vi "GUI Main.vi"() -> ()   [LabVIEW 2020]
uses:
  <vilib>/Instr/_visa.llb/VISA Configure Serial Port (Instr).vi
  <vilib>/picture/3D Picture Control/Object/Create Object (name).vi
  <vilib>/picture/3D Picture Control/NI_3D Picture Control.lvlib
panel:
  in  "Resource Name":refnum<visa-resource-name>="COM4"
  in  "Release":bool
  in  "Lock":bool
  in  "Jaw":bool
  in  "Stop":bool
  in  "1":dbl(knob) scale=-30.0..10.0
  in  "2":dbl(knob) scale=-70.0..-15.0
  in  "0":dbl(knob)
  out "Robotic Arm Simulation":refnum<vi>(3d-picture)
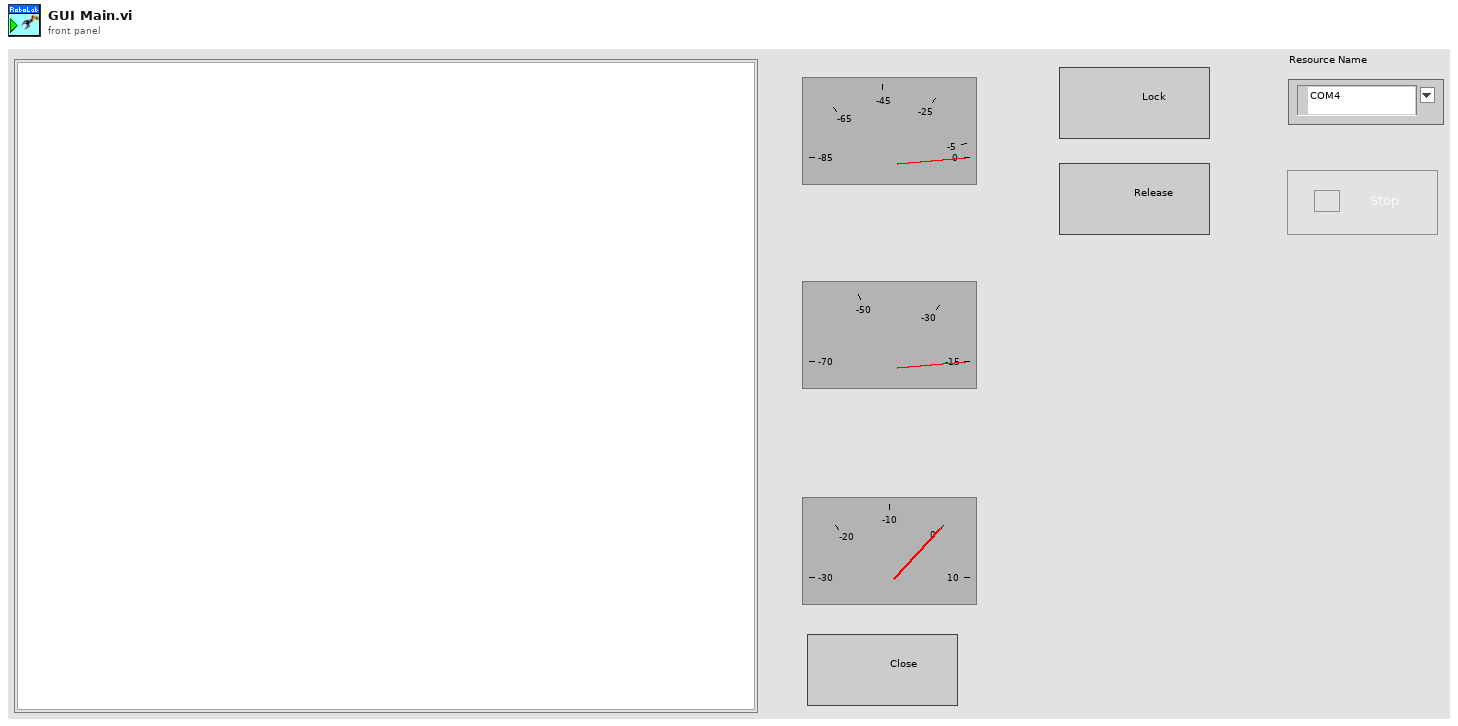
[diagram p1: front panel]
types:
  T1 = cluster{"Red":sgl, "Green":sgl, "Blue":sgl, "Alpha":sgl}
  T2 = cluster{"Name":string, "Parent":string, "Type":enum16{"Joint", "Box", "Cylinder", "Cone", "Sphere", "ASE File", "VRML File", "STL File", "Space"}, "Visible?":bool, "Geometry Definition":dbl[], "Position WRT Parent (X,Y,Z)":dbl[], "Rotation WRT Parent (degrees)":dbl[], "Joint Type":enum16{"Trans_X", "Trans_Y", "Trans_Z", "Rot_X", "Rot_Y", "Rot_Z", "None"}, "Geometry File Path":path, "Indent Level":i32, "Color":u32}[]
  T3 = cluster{"Joint Refnum":refnum<vi>, "Joint Type":enum16{"Trans_X", "Trans_Y", "Trans_Z", "Rot_X", "Rot_Y", "Rot_Z", "None"}, "Position WRT Parent":dbl[], "Rotation WRT Parent":dbl[], "Bar Refnum":refnum<vi>}[]
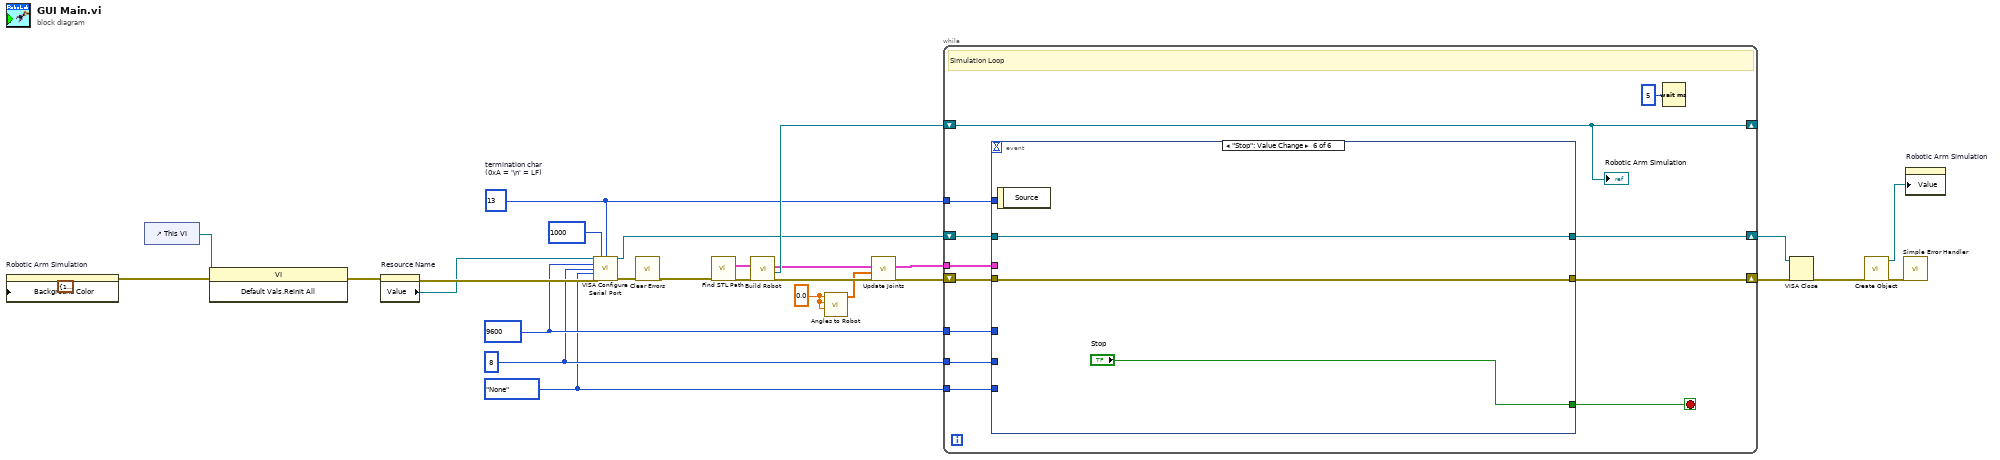
[diagram p0: block diagram]
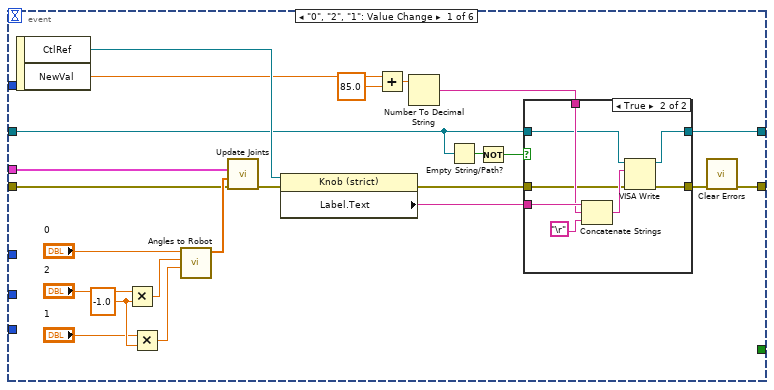
[diagram p2: hidden frame]
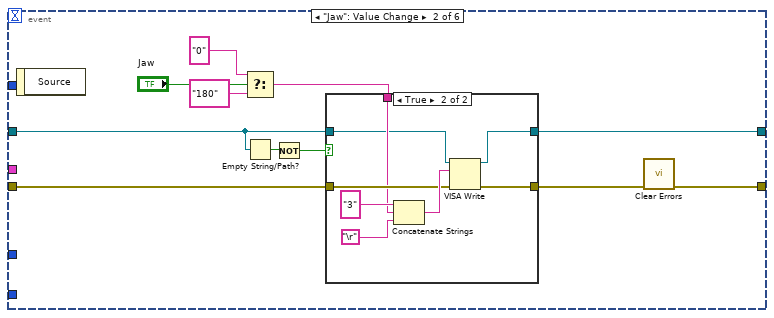
[diagram p4: hidden frame]
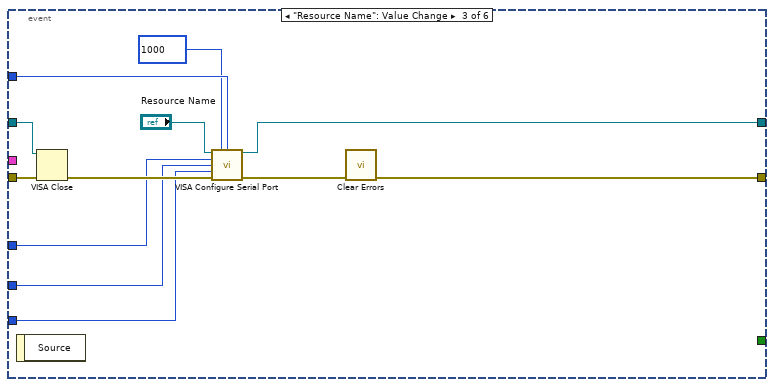
[diagram p6: hidden frame]
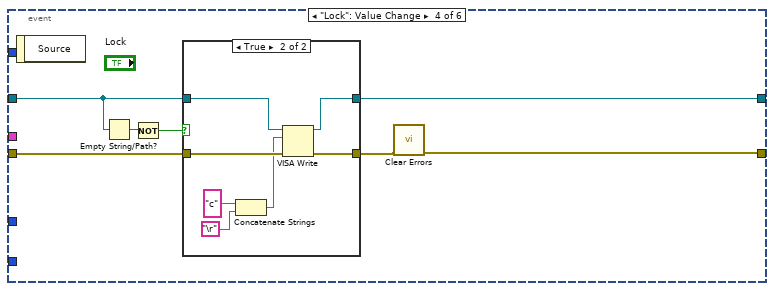
[diagram p7: hidden frame]
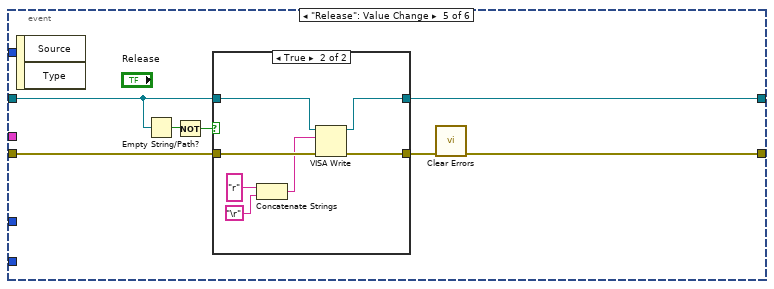
[diagram p9: hidden frame]
diagram:
  w4 = enum16{"None", "Odd", "Even", "Mark", "Space"}."None" ("parity (0:none)")
  w5 = u16 8 ("data bits (8)")
  w6 = u32 9600 ("baud rate (9600)")
  w7 = u8 13  # termination char (0xA = '\n' = LF)
  w18 = 0.0 ("Joint 0")
  n1 = property on="Robotic Arm Simulation" class="SceneGraphDisp (strict)"("Background Color"=T1 {"Red"=1.0, "Green"=1.0, "Blue"=1.0, "Alpha"=1.0}) -> (error out=w16:errorcluster)  [unwired: 2 in, 1 out]
  n2 = control-ref of="This VI"() -> (w15:refnum<vi>)
  n3 = invoke class="VI" method="Default Vals.Reinit All"(reference=w15, error in=w16) -> (error out=w10:errorcluster)  [unwired: 1 in, 2 out]
  n4 = property on="Resource Name" class="VISAName"(error in=w10) -> (error out=w9:errorcluster, "Value"=w8:refnum<visa-resource-name>)  [unwired: 1 in, 1 out]
  n5 = call-poly "VISA Configure Serial Port"("VISA resource name"=w8, "timeout (10sec)"=u32 1000, "termination char\n(0xA = '\\n' = LF)"=w7, "baud rate (9600)"=w6, "data bits (8)"=w5, "parity (0:none)"=w4, "error in (no error)"=w9) -> ("VISA resource name out"=w14:refnum<visa-resource-name>, "error out"=w3:errorcluster)  [unwired: 7 in]
  n6 = call <vilib>:"Clear Errors.vi"("error in (no error)"=w3) -> ("error out"=w2:errorcluster)  [unwired: 5 in, 1 out]
  n7 = call "Find STL Path.vi"("Error In"=w2) -> ("Error Out"=w26:errorcluster, "Array for myRoboLab Parts"=w25:T2)  [unwired: 9 in]
  n8 = call "Build Robot.vi"("error in"=w26, "Robotic Parts"=w25) -> ("error out"=w20:errorcluster, "Scene Out"=w24:refnum<vi>, "Joint Array"=w21:T3)  [unwired: 7 in]
  n9 = call "Angles to Robot.vi"("Joint 2"=w18, "Joint 1"=w18, "Joint 0"=w18) -> ("Angle array radians"=w17:dbl[])  [unwired: 7 in, 1 out]
  n10 = call "Update Joints.vi"("error in (no error)"=w20, "Joints"=w17, "Joint Array"=w21) -> ("error out"=w19:errorcluster)  [unwired: 8 in]
  n11 = while {
    tunnel: w21 -> [w39]
    shift-right: [w35] -> _
    shift-left: w24 -> [w35]
    shift-right: [w37] -> w13
    shift-left: w19 -> [w38]
    shift-right: [w32] -> w11
    shift-left: w14 -> [w33]
    tunnel: w7 -> [w31]
    tunnel: w6 -> [w30]
    tunnel: w5 -> [w29]
    tunnel: w4 -> [w28]
    stop <- w34 stop-if-true
    # "Simulation Loop"
    n12 = event shown="[5] \"Stop\": Value Change" {
      selector: _ -> [_ _ _ _ _ _]
      dyn-events: _ -> [_ _ _ _ _ _]
      timeout: _ -> [_ _ _ _ _ _]
      tunnel: w39 -> [w60 _ _ _ _ _]
      tunnel: w38 -> [w59 w83 w105 w112 w128 w139]
      tunnel: [w43 w76 w95 w109 w125 w139] -> w37
      tunnel: [_ _ _ _ _ "Stop"] -> w34
      tunnel: w33 -> [w41 w74 w104 w108 w123 w138]
      tunnel: [w50 w82 w101 w111 w127 w138] -> w32
      tunnel: w31 -> [_ _ w100 _ _ _]
      tunnel: w30 -> [_ _ w99 _ _ _]
      tunnel: w29 -> [_ _ w98 _ _ _]
      tunnel: w28 -> [_ _ w97 _ _ _]
      event "0", "2", "1": Value Change {
        w47 = -1.0 ("y")
        n13 = event-data() -> ("CtlRef"=w58:refnum<vi>, "NewVal"=w56:dbl)  [unwired: 1 in]
        n14 = Multiply(x="2", y=w47) -> (x*y=w48:dbl)
        n15 = Multiply(x="1", y=w47) -> (x*y=w45:dbl)
        n16 = call "Angles to Robot.vi"("Joint 2"=w45, "Joint 1"=w48, "Joint 0"="0") -> ("Angle array radians"=w62:dbl[])  [unwired: 7 in, 1 out]
        n17 = call "Update Joints.vi"("error in (no error)"=w59, "Joints"=w62, "Joint Array"=w60) -> ("error out"=w57:errorcluster)  [unwired: 8 in]
        n18 = property class="Knob (strict)"(reference=w58, error in=w57) -> (error out=w51:errorcluster, "Label.Text"=w54:string)  [unwired: 1 out]
        n19 = Add(x=w56, y=85.0) -> (x+y=w53:dbl)
        n20 = Number To Decimal String(number=w53) -> (decimal integer string=w52:string)  [unwired: 1 in]
        n21 = Empty String/Path?(string/path=w41) -> (empty?=w42:bool)
        n22 = Not(x=w42) -> (.not. x?=w40:bool)
        n23 = case shown="True" w40 {
          tunnel: w54 -> [_ w71]
          tunnel: w52 -> [_ w70]
          tunnel: w51 -> [w63 w68]
          tunnel: [w64 w67] -> w50
          tunnel: [w63 w66] -> w44
          tunnel: w41 -> [w64 w65]
          frame False {
          }
          frame True {
            n24 = Concatenate Strings(w71, w70, "\r") -> (w72:string)
            n25 = VISA Write(VISA resource name=w65, write buffer=w72, error in (no error)=w68) -> (VISA resource name out=w67:refnum<visa-resource-name>, error out=w66:errorcluster)  [unwired: 1 out]
          }
        }
        n26 = call <vilib>:"Clear Errors.vi"("error in (no error)"=w44) -> ("error out"=w43:errorcluster)  [unwired: 5 in, 1 out]
      }
      event "Jaw": Value Change {
        n27 = event-data() -> ()  [unwired: 1 in, 1 out]
        n28 = Select(t="0", s="Jaw", f="180") -> (s? t:f=w78:string)
        n29 = Empty String/Path?(string/path=w74) -> (empty?=w75:bool)
        n30 = Not(x=w75) -> (.not. x?=w73:bool)
        n31 = case shown="True" w73 {
          tunnel: w83 -> [w84 w92]
          tunnel: [w85 w91] -> w82
          tunnel: w78 -> [_ w89]
          tunnel: [w84 w87] -> w77
          tunnel: w74 -> [w85 w86]
          frame False {
          }
          frame True {
            n32 = Concatenate Strings("3" ("string"), w89, "\r") -> (w93:string)
            n33 = VISA Write(VISA resource name=w86, write buffer=w93, error in (no error)=w92) -> (VISA resource name out=w91:refnum<visa-resource-name>, error out=w87:errorcluster)  [unwired: 1 out]
          }
        }
        n34 = call <vilib>:"Clear Errors.vi"("error in (no error)"=w77) -> ("error out"=w76:errorcluster)  [unwired: 5 in, 1 out]
      }
      event "Resource Name": Value Change {
        n35 = event-data() -> ()  [unwired: 1 in, 1 out]
        n36 = VISA Close(VISA resource name=w104, error in (no error)=w105) -> (error out=w103:errorcluster)
        n37 = call-poly "VISA Configure Serial Port"("VISA resource name"="Resource Name", "timeout (10sec)"=u32 1000, "termination char\n(0xA = '\\n' = LF)"=w100, "baud rate (9600)"=w99, "data bits (8)"=w98, "parity (0:none)"=w97, "error in (no error)"=w103) -> ("VISA resource name out"=w101:refnum<visa-resource-name>, "error out"=w96:errorcluster)  [unwired: 7 in]
        n38 = call <vilib>:"Clear Errors.vi"("error in (no error)"=w96) -> ("error out"=w95:errorcluster)  [unwired: 5 in, 1 out]
      }
      event "Lock": Value Change {
        n39 = event-data() -> ()  [unwired: 1 in, 1 out]
        n40 = Empty String/Path?(string/path=w108) -> (empty?=w107:bool)
        n41 = Not(x=w107) -> (.not. x?=w106:bool)
        n42 = case shown="True" w106 {
          tunnel: w112 -> [w113 w121]
          tunnel: [w114 w120] -> w111
          tunnel: [w113 w116] -> w110
          tunnel: w108 -> [w114 w115]
          frame False {
          }
          frame True {
            n43 = Concatenate Strings("c" ("write buffer"), "\r") -> (w117:string)
            n44 = VISA Write(VISA resource name=w115, write buffer=w117, error in (no error)=w121) -> (VISA resource name out=w120:refnum<visa-resource-name>, error out=w116:errorcluster)  [unwired: 1 out]
          }
        }
        n45 = call <vilib>:"Clear Errors.vi"("error in (no error)"=w110) -> ("error out"=w109:errorcluster)  [unwired: 5 in, 1 out]
      }
      event "Release": Value Change {
        n46 = event-data() -> ()  [unwired: 1 in, 2 out]
        n47 = Empty String/Path?(string/path=w123) -> (empty?=w124:bool)
        n48 = Not(x=w124) -> (.not. x?=w122:bool)
        n49 = case shown="True" w122 {
          tunnel: w128 -> [w129 w137]
          tunnel: [w130 w136] -> w127
          tunnel: [w129 w132] -> w126
          tunnel: w123 -> [w130 w131]
          frame False {
          }
          frame True {
            n50 = Concatenate Strings("r" ("write buffer"), "\r") -> (w133:string)
            n51 = VISA Write(VISA resource name=w131, write buffer=w133, error in (no error)=w137) -> (VISA resource name out=w136:refnum<visa-resource-name>, error out=w132:errorcluster)  [unwired: 1 out]
          }
        }
        n52 = call <vilib>:"Clear Errors.vi"("error in (no error)"=w126) -> ("error out"=w125:errorcluster)  [unwired: 5 in, 1 out]
      }
      event "Stop": Value Change {
        n53 = event-data() -> ()  [unwired: 1 in, 1 out]
      }
    }
    n54 = Wait (ms)(milliseconds to wait=u32 5) -> ()  [unwired: 1 out]
    "Robotic Arm Simulation" <- w35
  }
  n55 = VISA Close(VISA resource name=w11, error in (no error)=w13) -> (error out=w12:errorcluster)
  n56 = call-poly <vilib>:"Create Object.vi"("error in (no error)"=w12) -> ("error out"=w23:errorcluster, "Scene:New Object"=w22:refnum<vi>)  [unwired: 9 in]
  n57 = call <vilib>:"Simple Error Handler.vi"("error in (no error)"=w23) -> ()  [unwired: 4 in, 5 out]
  n58 = property on="Robotic Arm Simulation" class="SceneGraphDisp (strict)"("Value"=w22) -> ()  [unwired: 2 in, 2 out]
